vi "倒计时系统.vi"() -> ()   [LabVIEW 2017]
panel:
  in  "停止":bool
  out "倒计时":string
  out "布尔":bool
  in  "开始倒计时":bool
  in  "定时时间选择":enum16{"20秒", "10秒", "6秒"}(ring)
  # "倒 计 时 器"
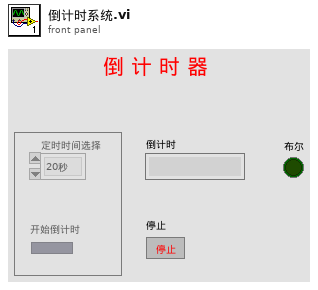
[diagram p1: front panel]
types:
  T1 = enum8{"Enabled", "Disabled", "Disabled and Grayed Out"}
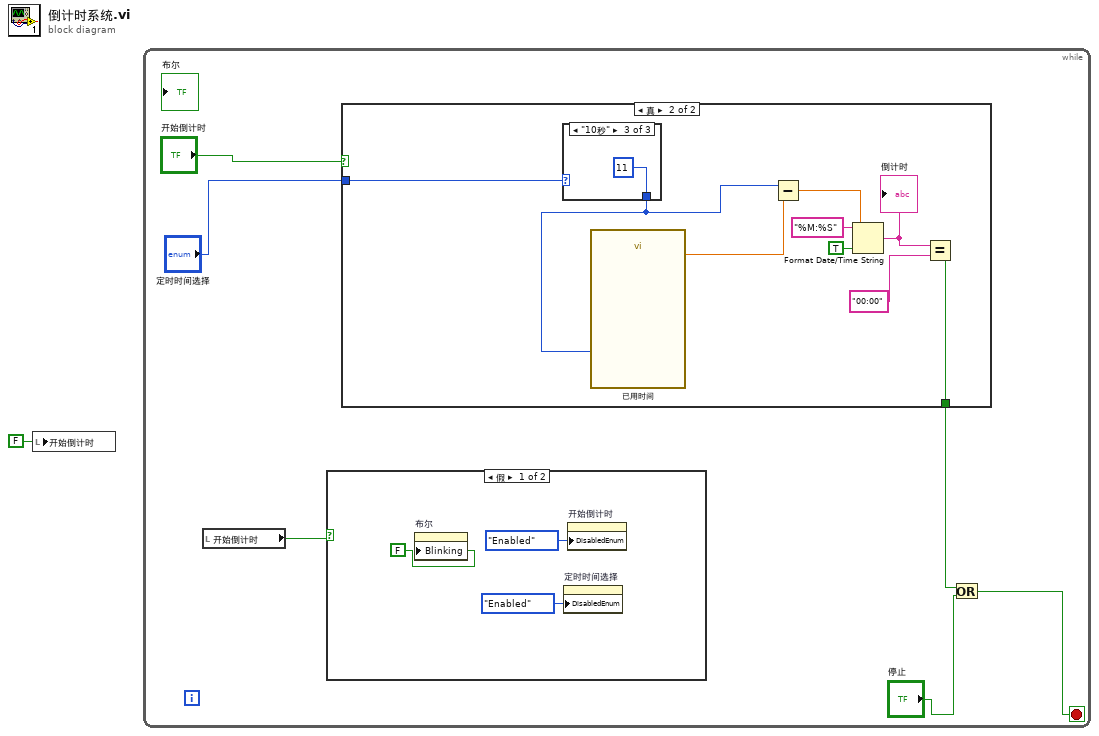
[diagram p0: block diagram]
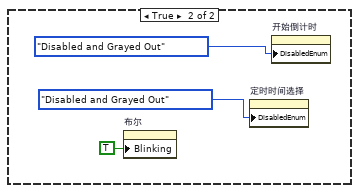
[diagram p2: hidden frame]
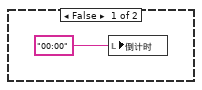
[diagram p3: hidden frame]
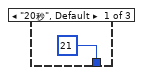
[diagram p4: hidden frame]
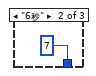
[diagram p5: hidden frame]
diagram:
  n1 = local write "开始倒计时"(FALSE ("开始倒计时")) -> ()
  n2 = while {
    stop <- w5 stop-if-true
    n3 = local read "开始倒计时"() -> (w3:bool)
    n4 = case shown="假" w3 {
      frame False {
        n5 = property on="布尔" class="Bool (严格)"("Blinking"=FALSE ("闪烁")) -> ()  [unwired: 2 in, 2 out]
        n6 = property on="定时时间选择" class="Enum (严格)"("DisabledEnum"=T1."Enabled" ("禁用")) -> ()  [unwired: 2 in, 2 out]
        n7 = property on="开始倒计时" class="Bool (严格)"("DisabledEnum"=T1."Enabled" ("禁用")) -> ()  [unwired: 2 in, 2 out]
      }
      frame True {
        n8 = property on="布尔" class="Bool (严格)"("Blinking"=TRUE ("闪烁")) -> ()  [unwired: 2 in, 2 out]
        n9 = property on="定时时间选择" class="Enum (严格)"("DisabledEnum"=T1."Disabled and Grayed Out" ("禁用")) -> ()  [unwired: 2 in, 2 out]
        n10 = property on="开始倒计时" class="Bool (严格)"("DisabledEnum"=T1."Disabled and Grayed Out" ("禁用")) -> ()  [unwired: 2 in, 2 out]
      }
    }
    n11 = case shown="真" "开始倒计时" {
      tunnel: [_ w18] -> w7
      tunnel: "定时时间选择" -> [_ w15]
      frame False {
        n12 = local write "倒计时"("00:00" ("日期/时间字符串")) -> ()
      }
      frame True {
        n13 = case shown="\"10秒\"" w15 {
          tunnel: [21 7 11] -> w16
          frame "20秒", Default {
          }
          frame "6秒" {
          }
          frame "10秒" {
          }
        }
        n14 = call "已用时间"("Time Target (s)"=w16) -> ("Elapsed Time (s)"=w17:dbl)  [unwired: 11 in, 7 out]
        n15 = Subtract(x=w16, y=w17) -> (x-y=w22:dbl)
        n16 = Format Date/Time String ("格式化日期/时间字符串")(time format string (%c)="%M:%S" ("时间格式字符串(%c)"), seconds (now)=w22, UTC format=TRUE ("UTC格式")) -> (date/time string=w20:string)
        "倒计时" <- w20
        n17 = Equal?(x=w20, y="00:00") -> (x = y?=w18:bool)
      }
    }
    n18 = Or(x=w7, y="停止") -> (x .or. y?=w5:bool)
  }
